vi "To String.vi"(8 "error in (no error)":errorcluster, 10 "Parameters":variant, 11 "Data1D in":refnum<class "Data1D.lvclass">) -> (0 "error out":errorcluster, 2 "String":string, 3 "Data1D out":refnum<class "Data1D.lvclass">)   [LabVIEW 2014, in "Data1D.lvclass"]
uses:
  Data1D.lvclass
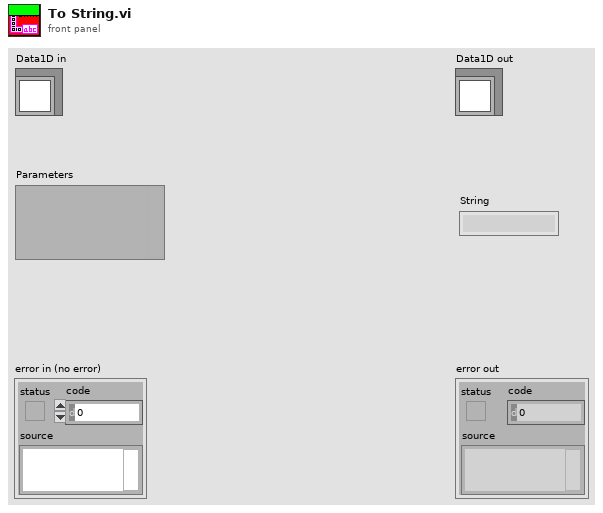
[diagram p1: front panel]
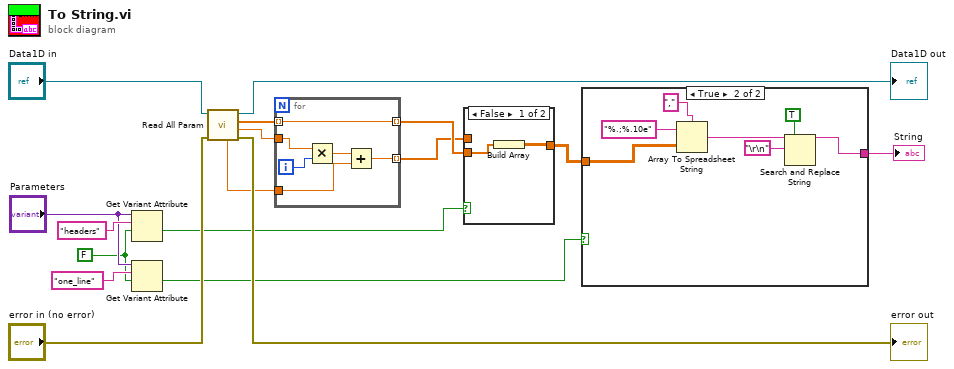
[diagram p0: block diagram]
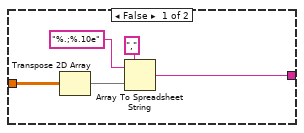
[diagram p2: hidden frame]
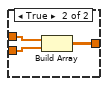
[diagram p3: hidden frame]
diagram:
  w4 = FALSE
  n1 = Get Variant Attribute(Variant="Parameters", name="headers", default value (empty Variant)=w4) -> (value=w3:bool)  [unwired: 1 in, 3 out]
  n2 = Get Variant Attribute(Variant="Parameters", name="one_line", default value (empty Variant)=w4) -> (value=w2:bool)  [unwired: 1 in, 3 out]
  n3 = call "Read All Param.vi"("error in (no error)"="error in (no error)", "Data1D in"="Data1D in") -> ("error out"=→"error out":errorcluster, "dt"=w14:dbl, "1D Array"=w15:dbl[], "Data1D out"=→"Data1D out":refnum<class "Data1D.lvclass">, "t0"=w1:dbl)  [unwired: 5 in]
  n4 = for {
    tunnel: w15 -> [w21] mode=indexing
    tunnel: w14 -> [w23]
    tunnel: [w20] -> w8 mode=indexing
    tunnel: [w21] -> w9 mode=indexing
    tunnel: w1 -> [w19]
    i -> [w22]
    n5 = Multiply(x=w23, y=w22) -> (x*y=w18:dbl)
    n6 = Add(x=w18, y=w19) -> (x+y=w20:dbl)
  }
  n7 = case shown="False" w3 {
    tunnel: [w25 w28] -> w10
    tunnel: w9 -> [w24 w27]
    tunnel: w8 -> [_ w26]
    frame False {
      n8 = Build Array(w24) -> (w25:dbl[][])
    }
    frame True {
      n9 = Build Array(w26, w27) -> (w28:dbl[][])
    }
  }
  n10 = case shown="True" w2 {
    tunnel: [w33 w38] -> w11
    tunnel: w10 -> [w31 w39]
    frame False {
      n11 = Transpose 2D Array(2D array=w31) -> (transposed array=w30:dbl[][])
      n12 = Array To Spreadsheet String(delimiter (Tab)=",", array=w30, 3:"%.;%.10e" ("format string")) -> (spreadsheet string=w33:string)
    }
    frame True {
      n13 = Array To Spreadsheet String(delimiter (Tab)=",", array=w39, 3:"%.;%.10e" ("format string")) -> (spreadsheet string=w36:string)
      n14 = Search and Replace String(replace all?=TRUE ("replace all? (F)"), input string=w36, search string="\r\n") -> (result string=w38:string)  [unwired: 5 in, 3 out]
    }
  }
  "String" <- w11
